vi "Get Bit (U16).vi"(10 "Bit":u8, 11 "Number":u16 format="%.0x") -> (2 "Value":bool=TRUE, 3 "Number Out":u16 format="%.0x")   [LabVIEW 2019, in "Bits.lvlib"]
doc: "Returns the bit value of the bit in the passed in number."
uses:
  Bits.lvlib
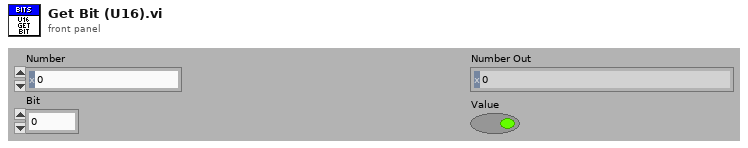
[diagram p1: front panel]
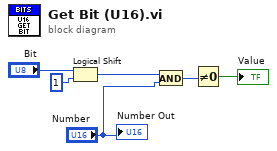
[diagram p0: block diagram]
diagram:
  n1 = Logical Shift(y="Bit", x=u16 1) -> (x << y=w4:u16)
  n2 = And(x=w4, y="Number") -> (x .and. y?=w2:u16)
  n3 = Not Equal To 0?(x=w2) -> (x != 0?=→"Value":bool)
  "Number Out" <- "Number"
